vi "EvaluateCollectionTriggerConditions.vi"(7 "dg_opState":string, 8 "error in":errorcluster, 9 "force trigger":bool, 10 "map":T2, 11 "OpStates in":variant) -> (0 "error out":errorcluster, 1 "collection type":T1, 2 "collect":bool, 3 "OpStates out":variant, 4 "reason":string)   [LabVIEW 2017, in "Trigger.lvlib"]
uses:
  <vilib>/addons/InsightCM/Devices/Shared/Common/Trigger/Trigger.lvlib
  <vilib>/addons/PointValueMap/controls/PointMap.ctl
  <vilib>/addons/InsightCM/Devices/Shared/Common/Trigger/controls/ConditionType.ctl
  <vilib>/addons/InsightCM/Devices/Shared/Common/DataEventCreator/controls/Reason.ctl
  <vilib>/addons/InsightCM/Devices/Shared/Common/DataEventCreator/DataEventCreator.lvlib
  <vilib>/addons/PointValueMap/PointValueMap.lvlib
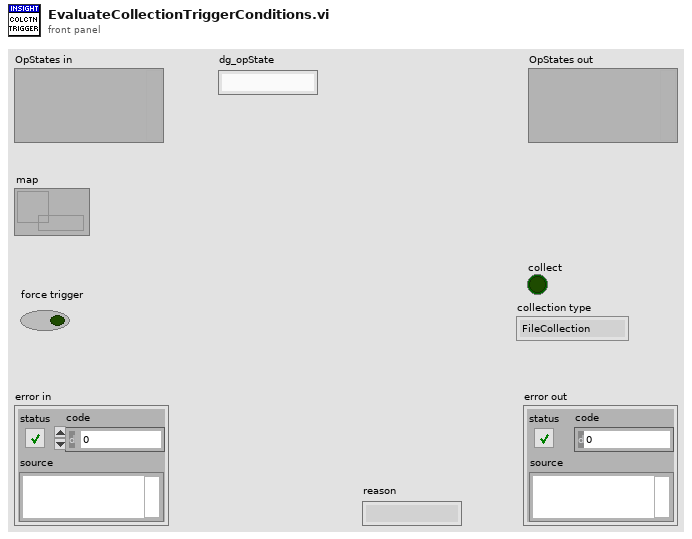
[diagram p1: front panel]
types:
  T1 = typedef "Trigger.lvlib/ConditionType.ctl" = enum16{"FileCollection", "TrendCollection"}
  T2 = typedef "PointValueMap.lvlib/PointMap.ctl" = refnum<data-value>
  T3 = typedef "DataEventCreator.lvlib/Reason.ctl" = enum16{"Periodic Event", "Delta EU Event", "Trend Event", "Alarm Event", "User Event", "Enter Operating State", "Exit Operating State", "Multiple Events", "Other"}
  T4 = typedef "Trigger.lvlib/TriggerCondition.ctl" = cluster{"Condition":T5, "LatchValue":string, "LatchTime":timestamp}
  T5 = typedef "Condition.ctl" = cluster{"Source":string, "Type":string, "Operator":string, "CompareTo":string, "DwellSeconds":dbl}
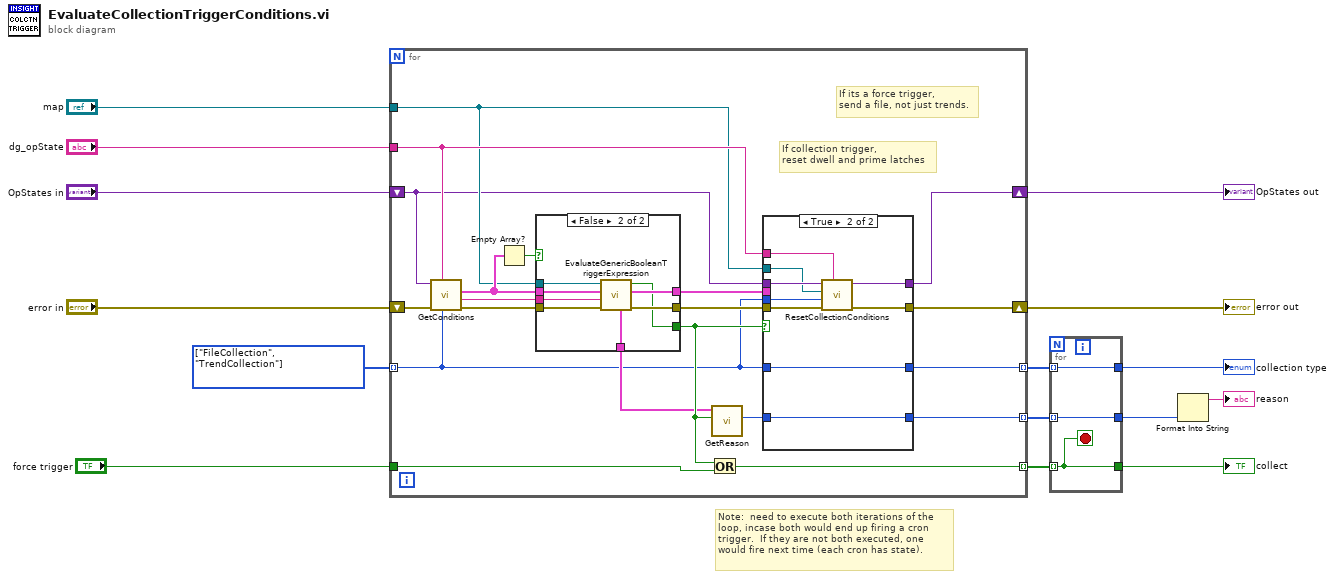
[diagram p0: block diagram]
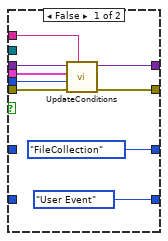
[diagram p2: hidden frame]
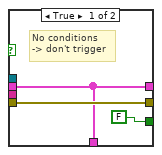
[diagram p3: hidden frame]
diagram:
  w9 = T1[] [enum."FileCollection", enum."TrendCollection"] items=["FileCollection", "TrendCollection"]
  # "Note:  need to execute both iterations of the\nloop, incase both would end up firing a cron\ntrigger.  If they are not both executed, one \nwould fire next time (each cron has state)."
  n1 = for {
    tunnel: [w20] -> w6 mode=indexing
    tunnel: "dg_opState" -> [w30]
    tunnel: "map" -> [w27]
    tunnel: w9 -> [w19] mode=indexing
    shift-right: [w28] -> w12
    shift-left: "OpStates in" -> [w25]
    shift-right: [w29] -> w13
    shift-left: "error in" -> [w26]
    tunnel: [w18] -> w7 mode=indexing
    tunnel: [w17] -> w5 mode=indexing
    tunnel: "force trigger" -> [w16]
    # "If its a force trigger,\nsend a file, not just trends."
    # "If collection trigger,\nreset dwell and prime latches"
    n2 = call <vilib>:"GetConditions.vi"("condition type"=w19, "dg_op"=w30, "error in (no error)"=w26, "operating states in"=w25) -> ("error out"=w34:errorcluster, "expression"=w35:string, "conditions"=w32:T4[])  [unwired: 4 in, 1 out]
    n3 = Empty Array?(array=w32) -> (empty?=w31:bool)
    n4 = case shown="False" w31 {
      tunnel: w35 -> [_ w64]
      tunnel: w34 -> [w55 w63]
      tunnel: [w55 w62] -> w33
      tunnel: [w54 w61] -> w24
      tunnel: w27 -> [_ w60]
      tunnel: [FALSE ("trigger") w59] -> w23
      tunnel: w32 -> [w54 w58]
      tunnel: [w54 w57] -> w22
      frame True {
        # "No conditions \n-> don't trigger"
      }
      frame False {
        n5 = call <vilib>:"EvaluateGenericBooleanTriggerExpression.vi"("error in (no error)"=w63, "expression"=w64, "all conditions"=w58, "map"=w60) -> ("error out"=w62:errorcluster, "all conditions out"=w61:T4[], "trigger"=w59:bool, "triggered conditions"=w57:T4[])  [unwired: 4 in]
      }
    }
    n6 = Or(x=w23, y=w16) -> (x .or. y?=w17:bool)
    n7 = call <vilib>:"GetReason.vi"("trigger"=w23, "triggered conditions"=w22) -> ("reason"=w21:T3)  [unwired: 9 in]
    n8 = case shown="True" w23 {
      tunnel: w33 -> [w44 w53]
      tunnel: w24 -> [w43 _]
      tunnel: w25 -> [w42 w51]
      tunnel: w19 -> [w41 w47]
      tunnel: w30 -> [w40 w48]
      tunnel: [w39 w52] -> w29
      tunnel: [w38 w50] -> w28
      tunnel: w27 -> [_ w49]
      tunnel: w21 -> [_ w46]
      tunnel: [Reason."User Event" ("Reason") w46] -> w20
      tunnel: [ConditionType."FileCollection" ("t") w45] -> w18
      tunnel: w19 -> [_ w45]
      frame False {
        n9 = call <vilib>:"UpdateConditions.vi"("ConditionType"=w41, "dg_op"=w40, "error in (no error)"=w44, "conditions"=w43, "operating states in"=w42) -> ("error out"=w39:errorcluster, "operating states out"=w38:variant)  [unwired: 5 in]
      }
      frame True {
        n10 = call <vilib>:"ResetCollectionConditions.vi"("dg_op"=w48, "error in (no error)"=w53, "ConditionType"=w47, "snapshot map"=w49, "operating states in"=w51) -> ("error out"=w52:errorcluster, "operating states out"=w50:variant)  [unwired: 5 in]
      }
    }
  }
  "error out" <- w13
  "OpStates out" <- w12
  n11 = for {
    tunnel: [w67] -> w4
    tunnel: w7 -> [w67] mode=indexing
    tunnel: [w66] -> w3
    tunnel: w6 -> [w66] mode=indexing
    tunnel: w5 -> [w65] mode=indexing
    tunnel: [w65] -> w2
    stop <- w65 stop-if-true
  }
  "collect" <- w2
  "collection type" <- w4
  n12 = Format Into String(w3) -> (resulting string=→"reason":string)  [unwired: 3 in, 1 out]
